vi "EPL-WavWrite.vi"(0 "path":path=path "C:/Experiment VIs/Utility VIs/Test VIs/test.wav", 1 "Fs (Hz)":dbl=100000.0, 5 "Data":dbl[](array[numeric]), 7 "Ref Name":string, 9 "Ref Val":dbl, 11 "error in (no error)":errorcluster) -> (4 "path out":path=path "C:/Experiment VIs/Utility VIs/Test VIs/test.wav", 15 "error out":errorcluster)   [LabVIEW 2020]
uses:
  <vilib>/sound2/lvsound2.llb/Sound Data Format.ctl
  <vilib>/Analysis/5stat.llb/RMS (DBL).vi
  <vilib>/sound2/lvsound2.llb/Sound File Write Open.vi
  <vilib>/sound2/lvsound2.llb/Sound File Write (DBL Single).vi
  <vilib>/Analysis/NI_AALPro.lvlib
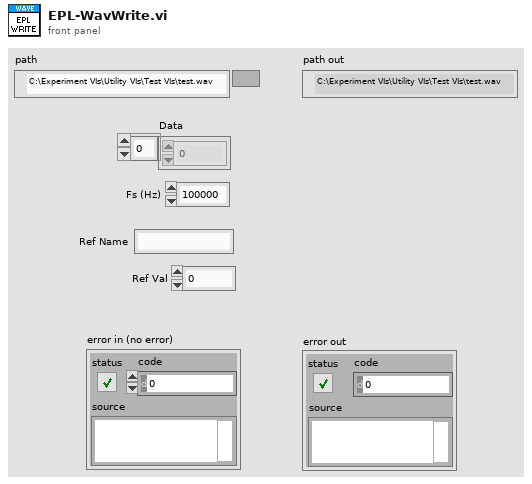
[diagram p1: front panel]
types:
  T1 = typedef "Sound Data Format.ctl" = cluster{"sample rate (S/s)":dbl, "number of channels":i32, "bits per sample":i32}
  T2 = enum16{"open", "replace", "create", "open or create", "replace or create", "replace or create with confirmation"}
  T3 = typedef "Sound File Refnum.ctl" = refnum<file>
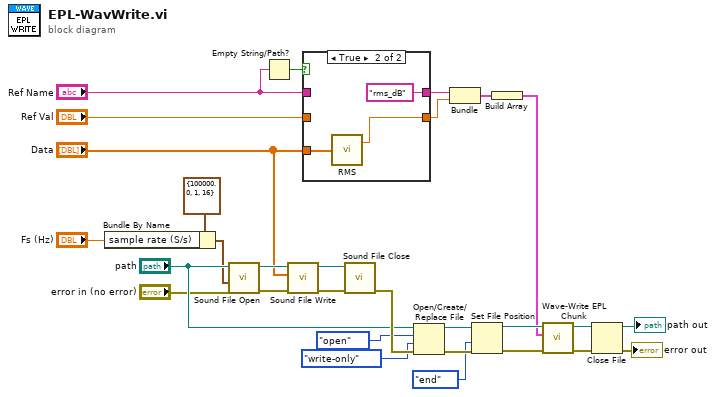
[diagram p0: block diagram]
diagram:
  n1 = Bundle By Name(cluster=T1 {"sample rate (S/s)"=100000.0, "number of channels"=1, "bits per sample"=16} ("sound format"), "sample rate (S/s)"="Fs (Hz)") -> (w9:T1)
  n2 = call-poly <vilib>:"Sound File Open.vi"("error in (no error)"="error in (no error)", "sound format"=w9, "path"="path") -> ("error out"=w29:errorcluster, "sound file refnum"=w28:T3)  [unwired: 7 in]
  n3 = Empty String/Path?(string/path="Ref Name") -> (empty?=w8:bool)
  n4 = call-poly <vilib>:"Sound File Write.vi"("error in (no error)"=w29, "data"="Data", "sound file refnum"=w28) -> ("error out"=w27:errorcluster, "sound file refnum out"=w25:T3)  [unwired: 7 in]
  n5 = case shown="True" w8 {
    tunnel: "Ref Name" -> [w31 _]
    tunnel: [w31 "rms_dB" ("Ref Name")] -> w4
    tunnel: [w30 w32] -> w3
    tunnel: "Ref Val" -> [w30 _]
    tunnel: "Data" -> [_ w33]
    frame False {
    }
    frame True {
      n6 = call-poly <vilib>:"RMS.vi"("X"=w33) -> ("rms value"=w32:dbl)  [unwired: 1 out]
    }
  }
  n7 = call <vilib>:"Sound File Close.vi"("error in (no error)"=w27, "sound file refnum"=w25) -> ("error out"=w26:errorcluster)  [unwired: 9 in]
  n8 = Open/Create/Replace File(file path (use dialog)="path", error in=w26, operation (0:open)=T2."open", access (0:read/write)=enum16{"read/write", "read-only", "write-only"}."write-only") -> (refnum out=w22:refnum<file>, error out=w23:errorcluster)  [unwired: 2 in, 1 out]
  n9 = Bundle("Ref Name"=w4, "rms value"=w3) -> (w2:cluster{"Ref Name":string, "rms value":dbl})  [unwired: 1 in]
  n10 = Set File Position(refnum=w22, from (0:start)=enum16{"start", "end", "current"}."end", error in=w23) -> (refnum out=w18:refnum<file>, error out=w17:errorcluster)  [unwired: 1 in]
  n11 = Build Array(w2) -> (w1:cluster{"Ref Name":string, "rms value":dbl}[])
  n12 = call "Wave-Write EPL Chunk.vi"("error in (no error)"=w17, "EPL Variables"=w1, "refnum"=w18) -> ("error out"=w16:errorcluster, "refnum out"=w15:refnum<file>)  [unwired: 7 in]
  n13 = Close File(refnum=w15, error in=w16) -> (path=→"path out":path, error out=→"error out":errorcluster)
